vi "version.vi"() -> ()   [LabVIEW 2010]
panel:
  out "VI path":path
  out "this version":path
  out "ceeserver version":timestamp
  out "This version":timestamp
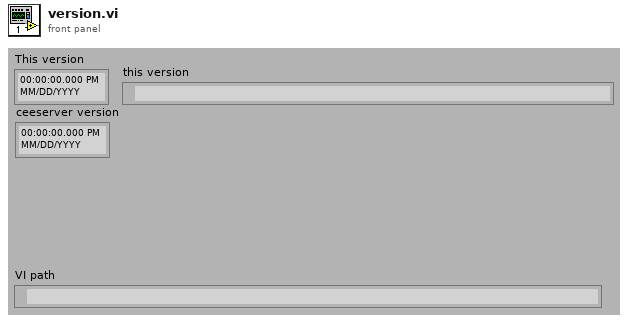
[diagram p1: front panel]
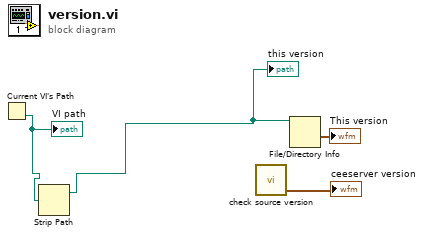
[diagram p0: block diagram]
diagram:
  n1 = Current VI's Path() -> (path=w3:path)
  "VI path" <- w3
  n2 = Strip Path(path=w3) -> (stripped path=w2:path)  [unwired: 1 out]
  "this version" <- w2
  n3 = call "check source version.vi"() -> ("time stamp"=→"ceeserver version":timestamp)  [unwired: 3 in, 1 out]
  n4 = File/Directory Info(path=w2) -> (last mod=→"This version":timestamp)  [unwired: 1 in, 6 out]
